vi "WaitAnswer.vi"(2 "error in (no error)":errorcluster, 3 "VISA resource name in":refnum<visa-resource-name>) -> (0 "error out":errorcluster, 1 "VISA resource name out":refnum<visa-resource-name>)   [LabVIEW 2016]
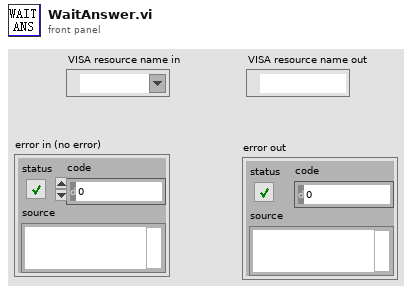
[diagram p1: front panel]
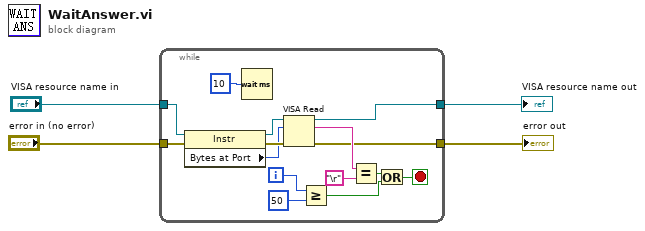
[diagram p0: block diagram]
diagram:
  n1 = while {
    tunnel: "VISA resource name in" -> [w14]
    tunnel: [w9] -> w3
    tunnel: "error in (no error)" -> [w6]
    tunnel: [w5] -> w1
    i -> [w18]
    stop <- w12 stop-if-true
    n2 = property class="Instr"(reference=w14, error in=w6) -> (reference out=w16:refnum<visa-resource-name>, error out=w15:errorcluster, "Bytes at Port"=w13:u32)
    n3 = Wait (ms)(milliseconds to wait=u32 10 ("等待时间（毫秒）")) -> ()  [unwired: 1 out]
    n4 = VISA Read(VISA resource name=w16, byte count=w13, error in (no error)=w15) -> (VISA resource name out=w9:refnum<visa-resource-name>, read buffer=w11:string, error out=w5:errorcluster)  [unwired: 1 out]
    n5 = Greater Or Equal?(x=w18, y=50) -> (x >= y?=w7:bool)
    n6 = Equal?(x=w11, y="\r") -> (x = y?=w8:bool)
    n7 = Or(x=w8, y=w7) -> (x .or. y?=w12:bool)
  }
  "VISA resource name out" <- w3
  "error out" <- w1
